vi "Actor Core.vi"(8 "error in":errorcluster, 11 "Generic Data Logger Card in":refnum<class "Generic Data Logger Card.lvclass">) -> (0 "error out":errorcluster, 3 "Actor out":refnum<class "Actor.lvclass">)   [LabVIEW 2013, in "Generic Data Logger.lvlib" / "Generic Data Logger Card.lvclass"]
doc: "(<B>Filename</B>: Actor Framework.lvlib:Actor.lvclass:Actor Core.vi)\n\nReceives messages to the actor, reacts to them, and initiates any error handling that may shut the actor down.\n\nDescendant classes may override this VI to append parallel tasks for the actor to complete while it handles messages. Overrides use the Call Parent Method node."
uses:
  Generic Data Logger Card.lvclass
  <vilib>/ActorFramework/Actor/Actor.lvclass
  Display Panel/Data Logger Display/Data Logger Display.lvclass
  Generic Instrument/Generic Card/Generic Card.lvclass/Generic Card.ctl
  Generic Instrument/Generic Card/Generic Card.lvclass
  <vilib>/ActorFramework/Actor/Actor.lvclass/Actor.ctl
  <vilib>/ActorFramework/Message Enqueuer/Message Enqueuer.lvclass/Message Enqueuer.ctl
  Display Panel/Abstract Display Messages/Write time digit Msg/Write time digit Msg.lvclass/Write time digit Msg.ctl
  <vilib>/ActorFramework/Message Enqueuer/Init from Existing Queue.vi
  <vilib>/ActorFramework/Message Enqueuer/Enqueue.vi
  <vilib>/ActorFramework/Message Priority Queue/Priority Enqueue.vi
  <vilib>/ActorFramework/Message Enqueuer/Message Enqueuer.lvclass
  Display Panel/Abstract Display Messages/Write time digit Msg/Write time digit Msg.lvclass
  <vilib>/ActorFramework/Stop Msg/Stop Msg.lvclass
  Generic Instrument/Generic Instrument.lvclass
panel:
  in  "Stop Bit":bool
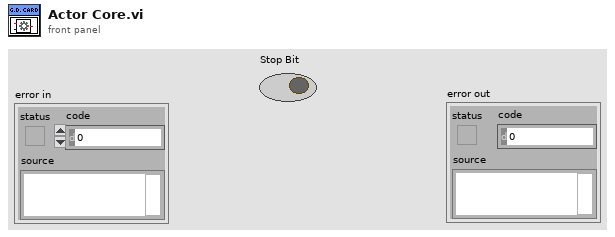
[diagram p1: front panel]
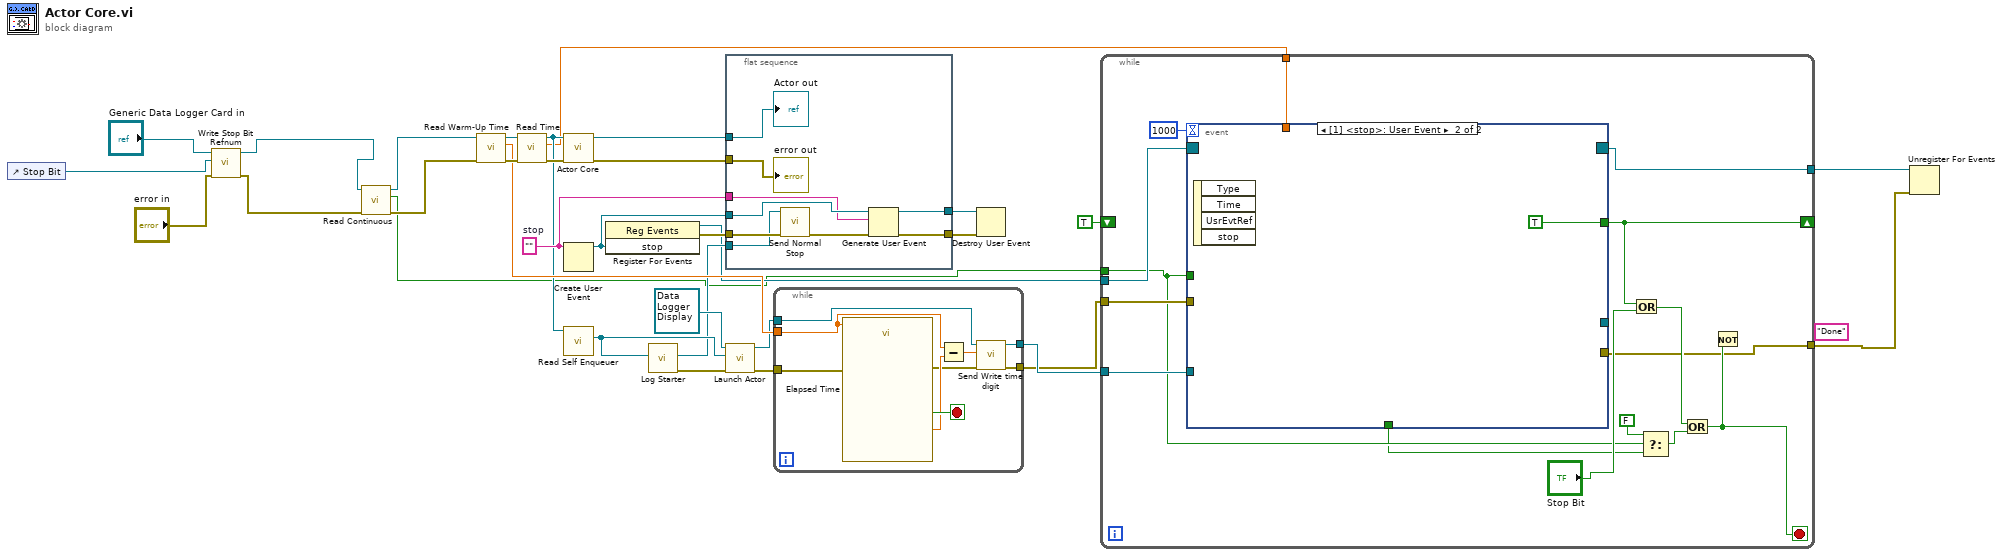
[diagram p0: block diagram]
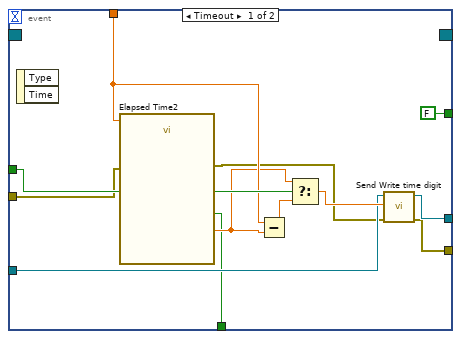
[diagram p2: hidden frame]
diagram:
  (unwired) "Done" ("Caption")
  w27 = ""  # stop
  n1 = control-ref of="Stop Bit"() -> (w6:refnum<vi>)
  n2 = call "Write Stop Bit Refnum.vi"("error in (no error)"="error in", "Stop Bit Refnum"=w6, "Generic Card in"="Generic Data Logger Card in") -> ("error out"=w4:errorcluster, "Generic Card out"=w7:refnum<class "Generic Data Logger Card.lvclass">)  [unwired: 7 in]
  n3 = call "Read Continuous.vi"("error in (no error)"=w4, "Generic Card in"=w7) -> ("error out"=w13:errorcluster, "Continuous?"=w11:bool, "Generic Card out"=w12:refnum<class "Generic Data Logger Card.lvclass">)  [unwired: 7 in]
  n4 = call "Read Warm-Up Time.vi"("error in (no error)"=w13, "Generic Card in"=w12) -> ("error out"=w25:errorcluster, "Warm-Up Time"=w23:dbl, "Generic Card out"=w26:refnum<class "Generic Data Logger Card.lvclass">)  [unwired: 7 in]
  n5 = call "Read Time .vi"("error in (no error)"=w25, "Generic Card in"=w26) -> ("error out"=w24:errorcluster, "Time"=w14:dbl, "Generic Card out"=w22:refnum<class "Generic Data Logger Card.lvclass">)  [unwired: 7 in]
  n6 = call-parent "Actor Core.vi"("error in"=w24, "Generic Card in"=w22) -> ("error out"=w33:errorcluster, "Actor out"=w32:refnum<class "Actor.lvclass">)  [unwired: 8 in]
  n7 = Create User Event(user event datatype=w27) -> (user event=w28:refnum<user-event>)  [unwired: 1 in, 1 out]
  n8 = call <vilib>:"Read Self Enqueuer.vi"("Actor"=w22) -> ("Self Enqueuer"=w18:refnum<class "Message Enqueuer.lvclass">)  [unwired: 10 in]
  n9 = register-events(w28) -> (reference out=w15:refnum<event-registration>, error out=w29:errorcluster)  [unwired: 2 in]
  n10 = call "Log Starter.vi"("Actor-to-Caller Enqueuer"=w18) -> ("error in"=w16:errorcluster, "Caller-To-Actor Enqueuer"=w17:refnum<class "Message Enqueuer.lvclass">)  [unwired: 9 in]
  n11 = flat-sequence {
    tunnel: w33 -> [w42]
    tunnel: w32 -> [w41]
    tunnel: [w40] -> w31
    tunnel: [w39] -> w30
    tunnel: w29 -> [w37]
    tunnel: w28 -> [w36]
    tunnel: w27 -> [w35]
    tunnel: w17 -> [w34]
    frame #0 {
      n12 = call <vilib>:"Send Normal Stop.vi"("error in (no error)"=w37, "Message Enqueuer"=w34) -> ("error out"=w38:errorcluster)  [unwired: 9 in]
      n13 = Generate User Event(user event=w36, event data cluster=w35, error in=w38) -> (user event out=w40:refnum<user-event>, error out=w39:errorcluster)  [unwired: 1 in]
      "error out" <- w42
      "Actor out" <- w41
    }
  }
  n14 = call <vilib>:"Launch Actor.vi"("error in (no error)"=w16, "Actor-to-Caller Enqueuer"=w18, "Actor"=refnum<class "Data Logger Display.lvclass"> refnum ("Display Panel.lvlib:Data Logger Display.lvclass")) -> ("error out"=w20:errorcluster, "Caller-To-Actor Enqueuer"=w21:refnum<class "Message Enqueuer.lvclass">)  [unwired: 7 in]
  n15 = while {
    tunnel: w23 -> [w51]
    tunnel: w21 -> [w46]
    tunnel: w20 -> [w45]
    tunnel: [w44] -> w10
    tunnel: [w43] -> w9
    stop <- w50 stop-if-true
    n16 = call "Elapsed Time"("Time Target (s)"=w51, "error in (no error)"=w45) -> ("Elapsed Time (s)"=w49:dbl, "Time has Elapsed"=w50:bool, "error out"=w47:errorcluster)  [unwired: 10 in, 5 out]
    n17 = Subtract(x=w51, y=w49) -> (x-y=w48:dbl)
    n18 = call "Send Write time digit.vi"("error in (no error)"=w47, "Time"=w48, "Message Enqueuer"=w46) -> ("error out"=w43:errorcluster, "Message Enqueuer out"=w44:refnum<class "Message Enqueuer.lvclass">)  [unwired: 7 in]
  }
  n19 = Destroy User Event(user event=w31, error in=w30) -> ()  [unwired: 1 out]
  n20 = while {
    tunnel: w15 -> [w58]
    tunnel: w14 -> [w65]
    tunnel: w11 -> [w57]
    tunnel: w10 -> [w64]
    tunnel: w9 -> [w63]
    shift-right: [w62] -> _
    shift-left: TRUE ("Stop Button") -> [_]
    tunnel: [w52] -> w1
    tunnel: [w53] -> w2
    stop <- w54 stop-if-true
    n21 = event shown="[1] <stop>: User Event" {
      selector: w58 -> [_ _]
      dyn-events: [_ _] -> w53
      timeout: 1000 -> [_ _]
      tunnel: w65 -> [w77 _]
      tunnel: w57 -> [w78 _]
      tunnel: w64 -> [w73 _]
      tunnel: w63 -> [w72 _]
      tunnel: [FALSE ("Stop Button") TRUE ("Stop Button")] -> w62
      tunnel: [w70 _] -> w55
      tunnel: [w69 _] -> _
      tunnel: [w68 _] -> w52
      event Timeout {
        n22 = event-data() -> ()  [unwired: 1 in, 2 out]
        n23 = call "Elapsed Time2"("Time Target (s)"=w77, "error in (no error)"=w72) -> ("Elapsed Time (s)"=w76:dbl, "Time has Elapsed"=w70:bool, "error out"=w71:errorcluster)  [unwired: 10 in, 5 out]
        n24 = Subtract(x=w77, y=w76) -> (x-y=w75:dbl)
        n25 = Select(t=w76, s=w78, f=w75) -> (s? t:f=w74:dbl)
        n26 = call "Send Write time digit.vi"("error in (no error)"=w71, "Time"=w74, "Message Enqueuer"=w73) -> ("error out"=w68:errorcluster, "Message Enqueuer out"=w69:refnum<class "Message Enqueuer.lvclass">)  [unwired: 7 in]
      }
      event User Event {
        n27 = event-data() -> ()  [unwired: 1 in, 4 out]
      }
    }
    n28 = Or(x=w62, y="Stop Bit") -> (x .or. y?=w59:bool)
    n29 = Select(t=FALSE ("f"), s=w57, f=w55) -> (s? t:f=w60:bool)
    n30 = Or(x=w59, y=w60) -> (x .or. y?=w54:bool)
    n31 = Not(x=w54) -> ()  [unwired: 1 out]
  }
  n32 = Unregister For Events(event registration refnum=w2, error in=w1) -> ()  [unwired: 1 out]
